vi "Decode VSM.vi"(11 "VSM Word":i16) -> (3 "Enum":T1)   [LabVIEW 2015]
uses:
  VSM States.ctl
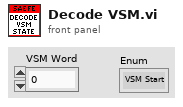
[diagram p1: front panel]
types:
  T1 = typedef "VSM States.ctl" = enum16{"VSM Start", "Pre-Charge Init", "Pre-Charge Active", "Pre-Charge Complete", "VSM Wait", "VSM Ready", "Motor Running", "Blink Fault Code", "Shutdown in Process", "Recycle Power"}
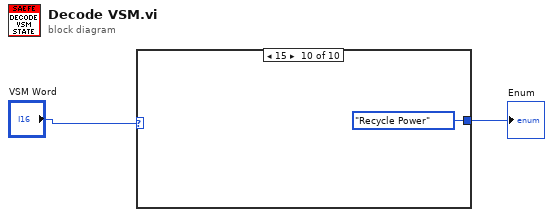
[diagram p0: block diagram]
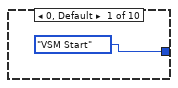
[diagram p2: hidden frame]
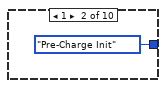
[diagram p3: hidden frame]
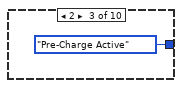
[diagram p4: hidden frame]
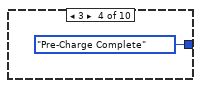
[diagram p5: hidden frame]
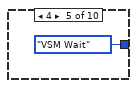
[diagram p6: hidden frame]
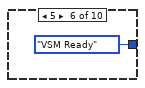
[diagram p7: hidden frame]
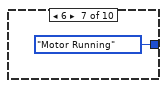
[diagram p8: hidden frame]
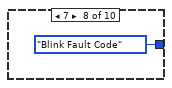
[diagram p9: hidden frame]
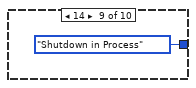
[diagram p10: hidden frame]
diagram:
  n1 = case shown="15" "VSM Word" {
    tunnel: [VSM_States."VSM Start" ("Enum") VSM_States."Pre-Charge Init" ("Enum") VSM_States."Pre-Charge Active" ("Enum") VSM_States."Pre-Charge Complete" ("Enum") VSM_States."VSM Wait" ("Enum") VSM_States."VSM Ready" ("Enum") VSM_States."Motor Running" ("Enum") VSM_States."Blink Fault Code" ("Enum") VSM_States."Shutdown in Process" ("Enum") VSM_States."Recycle Power" ("Enum")] -> w1
    frame 0, Default {
    }
    frame 1 {
    }
    frame 2 {
    }
    frame 3 {
    }
    frame 4 {
    }
    frame 5 {
    }
    frame 6 {
    }
    frame 7 {
    }
    frame 14 {
    }
    frame 15 {
    }
  }
  "Enum" <- w1
